vi "Get Current Buffer Index.vi"(8 "error in (no error)":errorcluster, 11 "Waveform Buffer in":refnum<class "Waveform Buffer.lvclass">) -> (0 "error out":errorcluster, 2 "Current Buffer Index":i32, 3 "Waveform Buffer out":refnum<class "Waveform Buffer.lvclass">)   [LabVIEW 2012, in "Waveform Data Logger Engine.lvlib" / "Waveform Buffer.lvclass"]
uses:
  Waveform Buffer.lvclass
  Waveform Buffer.lvclass/Waveform Buffer.ctl
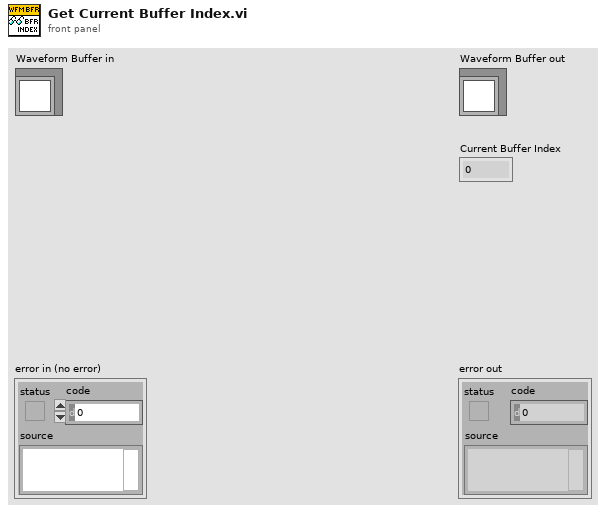
[diagram p1: front panel]
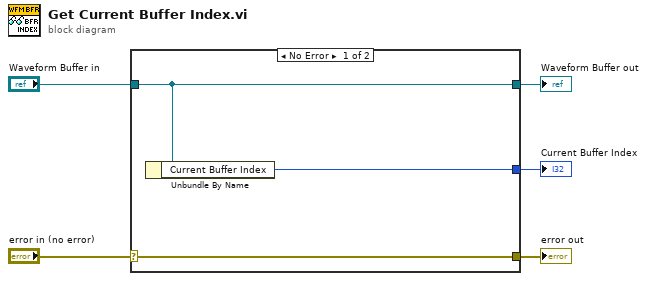
[diagram p0: block diagram]
diagram:
  n1 = case shown="No Error" "error in (no error)" {
    selector: "error in (no error)" -> [w8 w9]
    tunnel: [w8 w9] -> w4
    tunnel: [w7 w10] -> w2
    tunnel: "Waveform Buffer in" -> [w7 w10]
    tunnel: [w6 _] -> w1
    frame No Error {
      n2 = Unbundle By Name(w7) -> ("Current Buffer Index"=w6:i32)
    }
    frame Error {
    }
  }
  "error out" <- w4
  "Waveform Buffer out" <- w2
  "Current Buffer Index" <- w1
